vi "数据解析.vi"(11 "数组":u16[](array[numeric])=[16654, 1200, 17025, 780, 0, 58, 0, 19, 0, 385, 0, 15, 16744, 29677, 16759, 63517, 16550, 31242, 0, 134, 0, 130, 16979, 13107, 16979, 13107, 16979, 13107, 5888, 0, 1024, 0, 3, 1, 3, 1, 4, 0, 1, 0] format="%04xH") -> (2 "空闲":bool, 3 "综合生物毒性":T1={"时间"=timestamp(0 s since 1904-01-01), "水样测量结果"=0.0, "质控测量结果"=0.0, "R0"=0, "S0"=0, "Rt"=0, "St"=0, "CF"=0.0, "测量仓温度"=0.0, "培养仓温度"=0.0, "试剂余量"=0, "仪器状态"="", "空白结果"=0.0, "启动测量"=enum."启动水样测量", "停止测量"=FALSE})   [LabVIEW 2016, in "综合生物毒性.lvlib"]
panel:
  # "水样测量结果"
  # "质控测量结果"
  # "R0"
  # "S0"
  # "Rt"
  # "St"
  # "CF"
  # "培养仓温度"
  # "培养仓温度"
  # "试剂余量"
  # "仪器状态"
  # "因子编码"
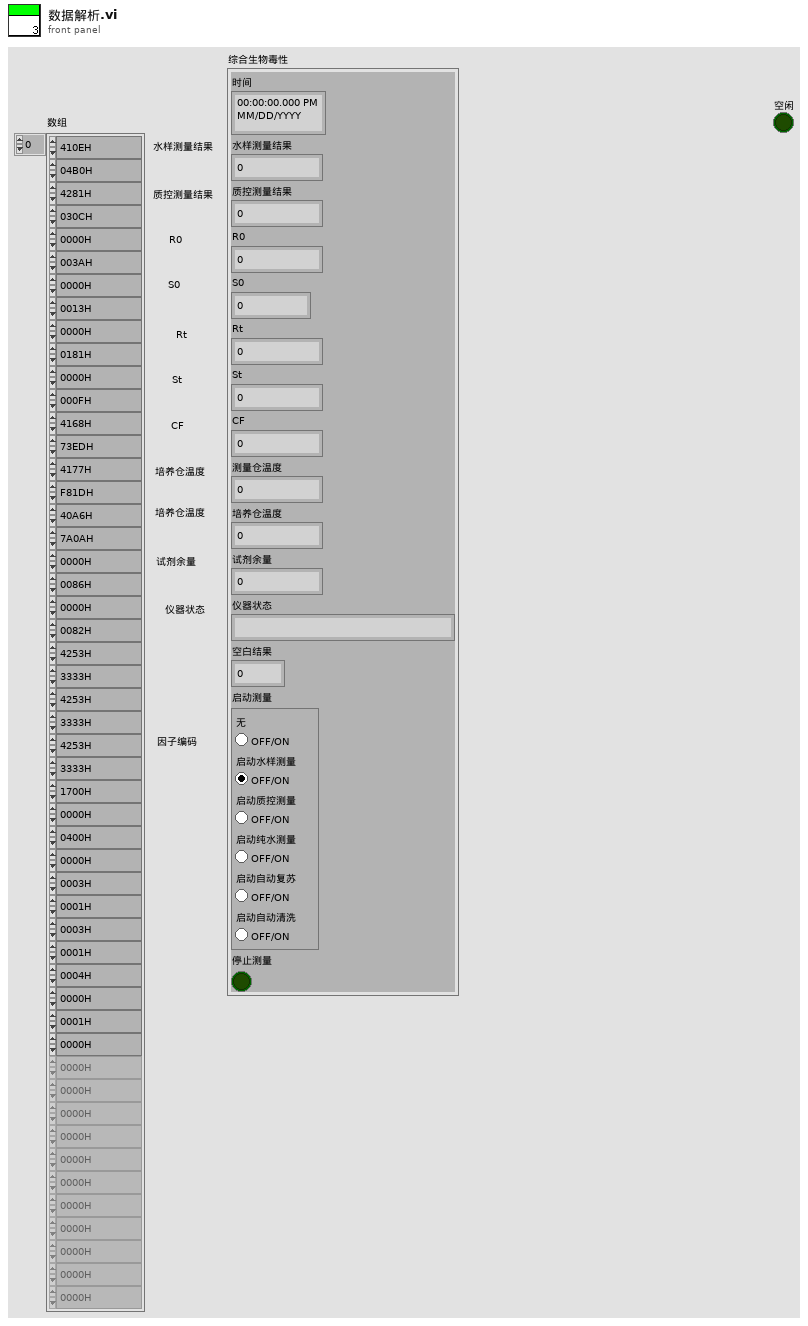
[diagram p1: front panel]
types:
  T1 = cluster{"时间":timestamp, "水样测量结果":sgl, "质控测量结果":sgl, "R0":i32, "S0":i32, "Rt":i32, "St":i32, "CF":sgl, "测量仓温度":sgl, "培养仓温度":sgl, "试剂余量":u32, "仪器状态":string, "空白结果":dbl, "启动测量":enum32{"无", "启动水样测量", "启动质控测量", "启动纯水测量", "启动自动复苏", "启动自动清洗"}, "停止测量":bool}
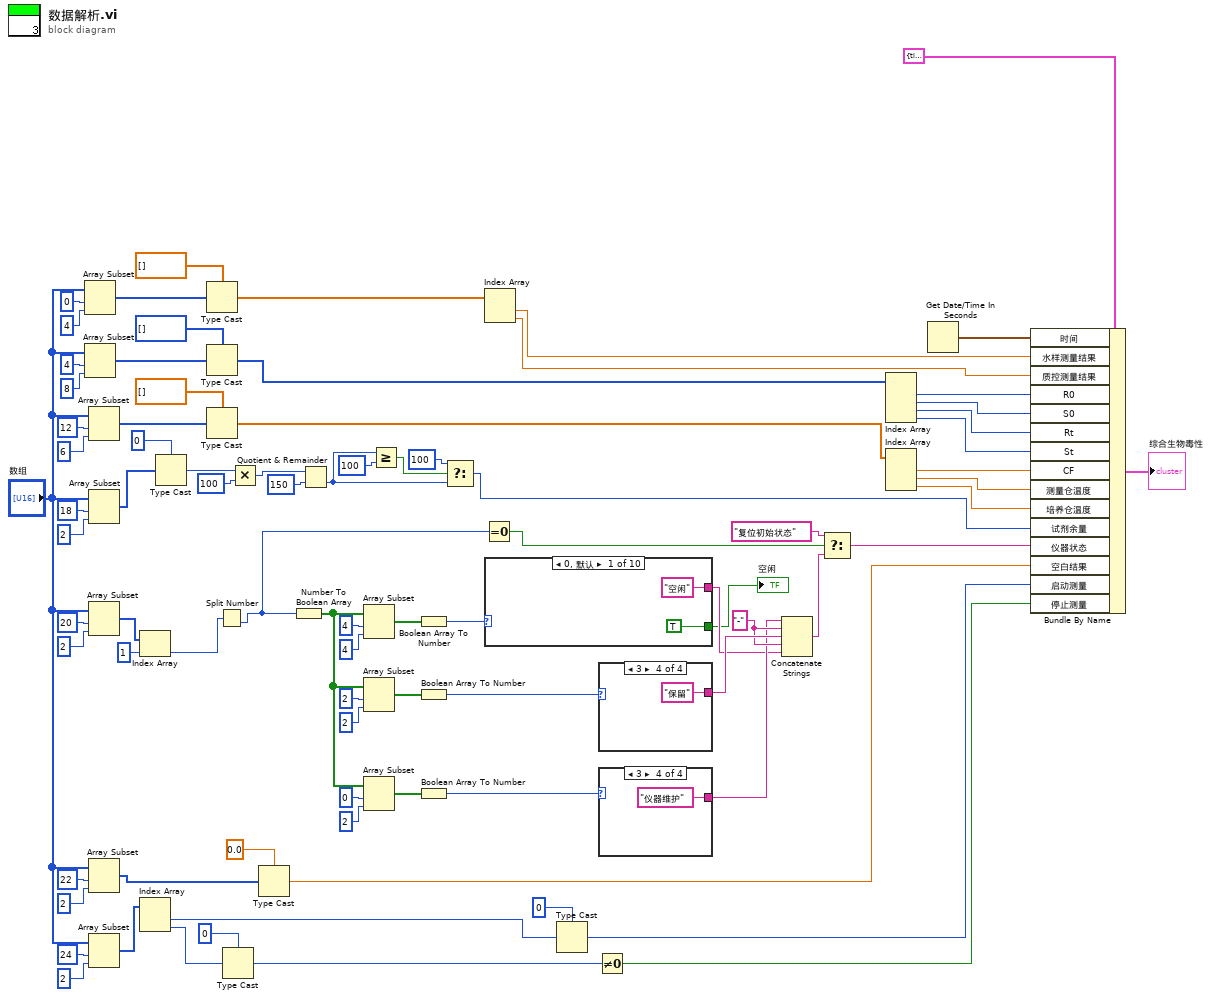
[diagram p0: block diagram]
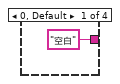
[diagram p2: hidden frame]
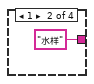
[diagram p3: hidden frame]
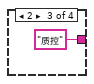
[diagram p4: hidden frame]
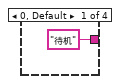
[diagram p5: hidden frame]
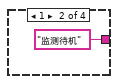
[diagram p6: hidden frame]
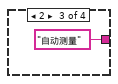
[diagram p7: hidden frame]
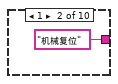
[diagram p8: hidden frame]
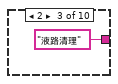
[diagram p9: hidden frame]
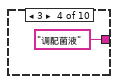
[diagram p10: hidden frame]
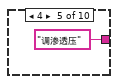
[diagram p11: hidden frame]
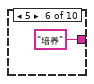
[diagram p12: hidden frame]
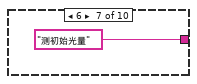
[diagram p13: hidden frame]
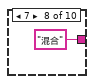
[diagram p14: hidden frame]
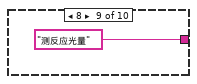
[diagram p15: hidden frame]
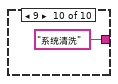
[diagram p16: hidden frame]
diagram:
  w32 = "-"
  n1 = Array Subset(array="数组", index=0 ("索引"), length=4 ("长度")) -> (w65:u16[])
  n2 = Array Subset(array="数组", index=4 ("索引"), length=8 ("长度")) -> (w60:u16[])
  n3 = Array Subset(array="数组", index=12 ("索引"), length=6 ("长度")) -> (w44:u16[])
  n4 = Array Subset(array="数组", index=18 ("索引"), length=2 ("长度")) -> (w46:u16[])
  n5 = Array Subset(array="数组", index=20 ("索引"), length=2 ("长度")) -> (w15:u16[])
  n6 = Array Subset(array="数组", index=22 ("索引"), length=2 ("长度")) -> (w9:u16[])
  n7 = Array Subset(array="数组", index=24 ("索引"), length=2 ("长度")) -> (w3:u16[])
  n8 = Index Array(array=w15, index=1 ("索引")) -> (element=w13:u16)
  n9 = Index Array(array=w3) -> (element #1=w51:u16, element #2=w2:u16)  [unwired: 2 in]
  n10 = Type Cast(type=u32 0, x=w46) -> (*(type *) &x=w35:u32)
  n11 = Type Cast(type=sgl[] [], x=w65) -> (*(type *) &x=w64:sgl[])
  n12 = Type Cast(type=i32[] [], x=w60) -> (*(type *) &x=w59:i32[])
  n13 = Type Cast(type=sgl[] [], x=w44) -> (*(type *) &x=w62:sgl[])
  n14 = Split Number(x=w13) -> (lo(x)=w12:u8)  [unwired: 1 out]
  n15 = Type Cast(type=i16 0 ("数字"), x=w2) -> (*(type *) &x=w49:i16)
  n16 = Multiply(x=w35, y=u32 100) -> (x*y=w39:u32)
  n17 = Type Cast(type=0.0, x=w9) -> (*(type *) &x=w4:dbl)
  n18 = Number To Boolean Array(number=w12) -> (Boolean array=w21:bool[])
  n19 = Quotient & Remainder(x=w39, y=u32 150) -> (floor(x/y)=w38:u32)  [unwired: 1 out]
  n20 = Array Subset(array=w21, index=4 ("索引"), length=4 ("长度")) -> (w29:bool[])
  n21 = Array Subset(array=w21, index=2 ("索引"), length=2 ("长度")) -> (w26:bool[])
  n22 = Array Subset(array=w21, index=0 ("索引"), length=2 ("长度")) -> (w20:bool[])
  n23 = Greater Or Equal?(x=w38, y=u32 100) -> (x >= y?=w36:bool)
  n24 = Boolean Array To Number(Boolean array=w29) -> (number=w25:u32)
  n25 = Boolean Array To Number(Boolean array=w26) -> (number=w24:u32)
  n26 = Boolean Array To Number(Boolean array=w20) -> (number=w19:u32)
  n27 = Select(t=u32 100 ("y"), s=w36, f=w38) -> (s? t:f=w41:u32)
  n28 = Equal To 0?(x=w12) -> (x = 0?=w18:bool)
  n29 = Index Array(array=w64) -> (element #1=w76:sgl, element #2=w75:sgl)  [unwired: 2 in]
  n30 = case shown="0, 默认" w25 {
    tunnel: ["空闲" "机械复位" "液路清理" "调配菌液" "调渗透压" "培养" "测初始光量" "混合" "测反应光量" "系统清洗"] -> w10
    tunnel: [TRUE _ _ _ _ _ _ _ _ _] -> w1
    frame 0, Default {
    }
    frame 1 {
    }
    frame 2 {
    }
    frame 3 {
    }
    frame 4 {
    }
    frame 5 {
    }
    frame 6 {
    }
    frame 7 {
    }
    frame 8 {
    }
    frame 9 {
    }
  }
  "空闲" <- w1
  n31 = Type Cast(type=i16 0 ("数字"), x=w51) -> (*(type *) &x=w52:i16)
  n32 = Not Equal To 0?(x=w49) -> (x != 0?=w54:bool)
  n33 = case shown="3" w24 {
    tunnel: ["空白" "水样" "质控" "保留"] -> w33
    frame 0, Default {
    }
    frame 1 {
    }
    frame 2 {
    }
    frame 3 {
    }
  }
  n34 = case shown="3" w19 {
    tunnel: ["待机" "监测待机" "自动测量" "仪器维护"] -> w11
    frame 0, Default {
    }
    frame 1 {
    }
    frame 2 {
    }
    frame 3 {
    }
  }
  n35 = Concatenate Strings(w11, w32, w33, w32, w10) -> (w16:string)
  n36 = Select(t="复位初始状态", s=w18, f=w16) -> (s? t:f=w7:string)
  n37 = Index Array(array=w59) -> (element #1=w74:i32, element #2=w73:i32, element #3=w72:i32, element #4=w71:i32)  [unwired: 4 in]
  n38 = Index Array(array=w62) -> (element #1=w70:sgl, element #2=w69:sgl, element #3=w68:sgl)  [unwired: 3 in]
  n39 = Get Date/Time In Seconds() -> (seconds since 1Jan1904=w67:timestamp)
  n40 = Bundle By Name(cluster=T1 {"时间"=timestamp(3782468077.4469967 s since 1904-01-01), "水样测量结果"=8.876144, "质控测量结果"=64.50595, "R0"=58, "S0"=19, "Rt"=385, "St"=15, "CF"=14.528302, "测量仓温度"=15.498075, "培养仓温度"=5.2023973, "试剂余量"=89, "仪器状态"="自动测量-空白-测反应光量", "空白结果"=0.0, "启动测量"=enum."启动自动清洗", "停止测量"=TRUE} ("综合生物毒性"), "时间"=w67, "水样测量结果"=w76, "质控测量结果"=w75, "R0"=w74, "S0"=w73, "Rt"=w72, "St"=w71, "CF"=w70, "测量仓温度"=w69, "培养仓温度"=w68, "试剂余量"=w41, "仪器状态"=w7, "空白结果"=w4, "启动测量"=w52, "停止测量"=w54) -> (→"综合生物毒性":T1)
